vi "Driver VI Template Name.vi"(11 "CD Template":refnum<class "NIVS_Inline Timing and Sync.lvclass">) -> (2 "Driver VI Template Name":string)   [LabVIEW 2020, in "NIVS_Inline Timing and Sync.lvclass"]
uses:
  NIVS_Inline Timing and Sync.lvclass
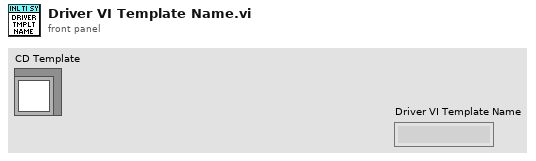
[diagram p1: front panel]
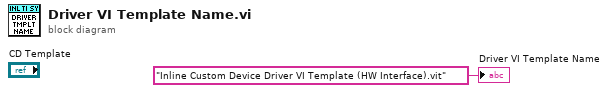
[diagram p0: block diagram]
diagram:
  "Driver VI Template Name" <- "Inline Custom Device Driver VI Template (HW Interface).vit" ("Driver VI Template Name")
